vi "Position Updated.vi"(8 "error in (no error)":errorcluster, 10 "New Position":dbl, 11 "Encoder Logic in":refnum<class "Encoder Logic.lvclass">) -> (0 "error out":errorcluster, 3 "Encoder Logic out":refnum<class "Encoder Logic.lvclass">)   [LabVIEW 2025, in "Encoder Logic.lvlib" / "Encoder Logic.lvclass"]
uses:
  Encoder Logic.lvclass
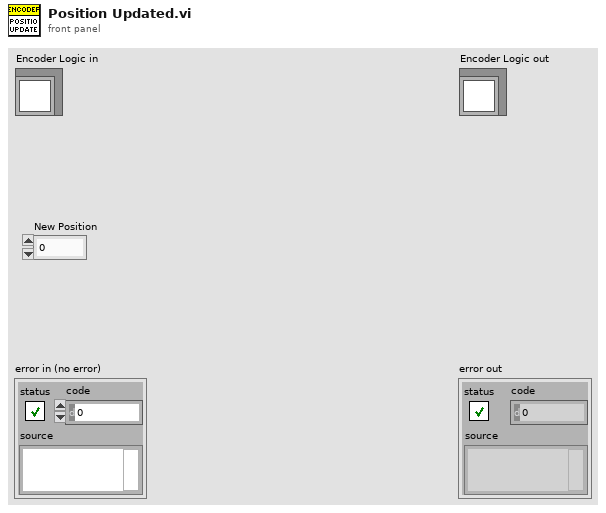
[diagram p1: front panel]
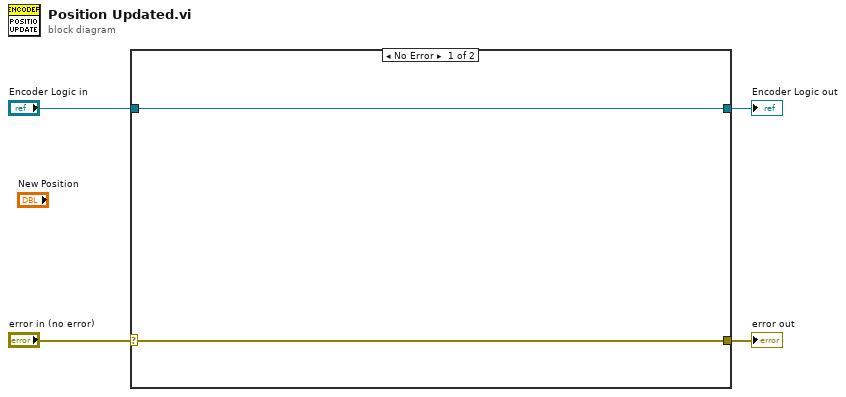
[diagram p0: block diagram]
diagram:
  n1 = case shown="No Error" "error in (no error)" {
    selector: "error in (no error)" -> [w5 w8]
    tunnel: [w5 w8] -> w3
    tunnel: [w6 w7] -> w1
    tunnel: "Encoder Logic in" -> [w6 w7]
    frame No Error {
    }
    frame Error {
    }
  }
  "error out" <- w3
  "Encoder Logic out" <- w1
